vi "Report Error.vi"(8 "error in (no error)":errorcluster, 11 "Class in":refnum<class "AB_UI_Frmwk_Installer.lvclass">) -> (0 "error out":errorcluster, 3 "Class out":refnum<class "AB_UI_Frmwk_Installer.lvclass">)   [LabVIEW 2020, in "AB_UI_Frmwk_Installer.lvclass"]
uses:
  <vilib>/AppBuilder/IB_Classes/Installer/UI/AB_UI_Frmwk_Installer.lvclass
  <resource>/Framework/Providers/Builds/AppBuilder/AB_UI_Frmwk.lvclass
  AppLibs/distkit/MDF/NI_MDF.lvlib
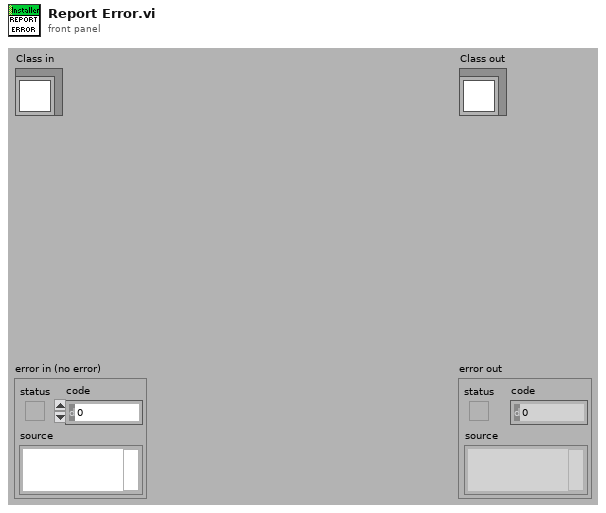
[diagram p1: front panel]
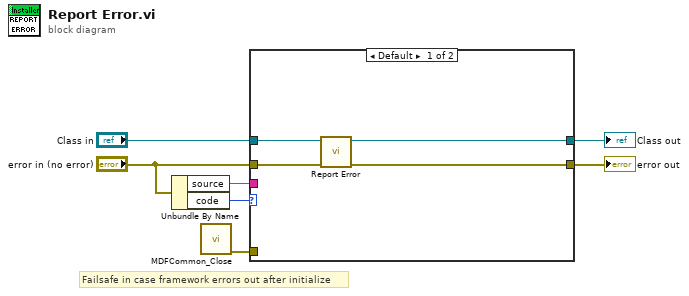
[diagram p0: block diagram]
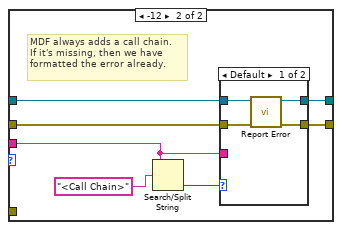
[diagram p2: hidden frame]
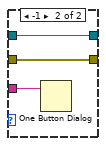
[diagram p3: hidden frame]
diagram:
  # "Failsafe in case framework errors out after initialize"
  n1 = Unbundle By Name("error in (no error)") -> ("source"=w6:string, "code"=w7:i32)
  n2 = call "MDFCommon_Close.vi"() -> ("error out"=w1:errorcluster)  [unwired: 11 in]
  n3 = case shown="Default" w7 {
    tunnel: w6 -> [_ w17]
    tunnel: "Class in" -> [w11 w15]
    tunnel: [w10 w14] -> w4
    tunnel: "error in (no error)" -> [w9 w13]
    tunnel: [w8 w12] -> w2
    tunnel: w1 -> [_ _]
    frame Default {
      n4 = call-parent "Report Error.vi"("error in (no error)"=w9, "AB_UI_Frmwk in"=w11) -> ("error out"=w8:errorcluster, "AB_UI_Frmwk out"=w10:refnum<class "AB_UI_Frmwk_Installer.lvclass">)  [unwired: 8 in]
    }
    frame -12 {
      # "MDF always adds a call chain.\nIf it's missing, then we have\nformatted the error already."
      n5 = Search/Split String(string=w17, search string/char (-)="<Call Chain>" ("string")) -> (offset of match=w16:i32)  [unwired: 3 out]
      n6 = case shown="Default" w16 {
        tunnel: w17 -> [_ w25]
        tunnel: w15 -> [w22 w24]
        tunnel: [w21 w24] -> w14
        tunnel: w13 -> [w20 w23]
        tunnel: [w19 w23] -> w12
        frame Default {
          n7 = call-parent "Report Error.vi"("error in (no error)"=w20, "AB_UI_Frmwk in"=w22) -> ("error out"=w19:errorcluster, "AB_UI_Frmwk out"=w21:refnum<class "AB_UI_Frmwk_Installer.lvclass">)  [unwired: 8 in]
        }
        frame -1 {
          n8 = One Button Dialog(message=w25) -> ()  [unwired: 1 in, 1 out]
        }
      }
    }
  }
  "error out" <- w2
  "Class out" <- w4
